vi "UDB_EN - Read.vi"(8 "error in":errorcluster, 11 "TSM Context Global Access in":refnum<class "TSM Context Data Access.lvclass">) -> (0 "error out":errorcluster, 2 "UDB_EN":bool[](array[boolean]), 3 "TSM Context Global Access out":refnum<class "TSM Context Data Access.lvclass">)   [LabVIEW 2019, in "TSM Context Data Access.lvclass"]
uses:
  TSM Context Data Access.lvclass
  TSM Context Data Access.lvclass/TSM Context Data Access.ctl
  <vilib>/NI_TestStand_SemiconductorModule/NI_TestStand_Semiconductor_Module.lvlibp
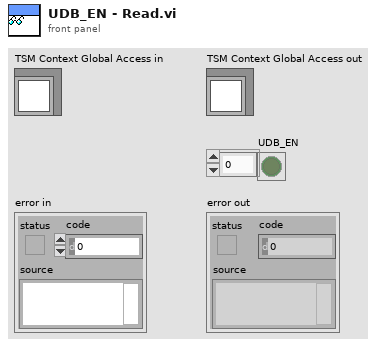
[diagram p1: front panel]
types:
  T1 = typedef "NI_TestStand_Semiconductor_Module.lvlibp/SemiconductorModuleContext.ctl" = refnum<k7>
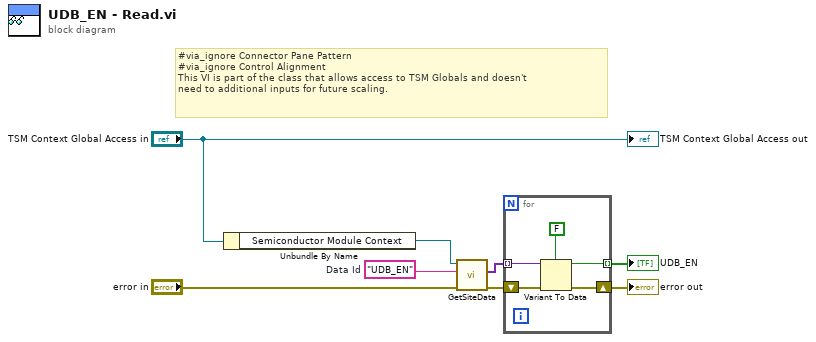
[diagram p0: block diagram]
diagram:
  w3 = "UDB_EN"  # Data Id
  # "#via_ignore Connector Pane Pattern\n#via_ignore Control Alignment \nThis VI is part of the class that allows access to TSM Globals and doesn't \nneed to additional inputs for future scaling."
  n1 = Unbundle By Name("TSM Context Global Access in") -> ("Semiconductor Module Context"=w4:T1)
  n2 = call <vilib>:"GetSiteData.vi"("error in (no error)"="error in", "Data Id"=w3, "Semiconductor Module Context"=w4) -> ("error out"=w5:errorcluster, "Site Data"=w2:variant[])  [unwired: 6 in, 1 out]
  n3 = for {
    tunnel: [w12] -> w1 mode=indexing
    tunnel: w2 -> [w10] mode=indexing
    shift-right: [w13] -> w7
    shift-left: w5 -> [w11]
    n4 = Variant To Data(error in=w11, type=FALSE, Variant=w10) -> (data=w12:bool, error out=w13:errorcluster)
  }
  "error out" <- w7
  "UDB_EN" <- w1
  "TSM Context Global Access out" <- "TSM Context Global Access in"
